vi "MC_ISM_main.vi"() -> ()   [LabVIEW 2017]
doc: "Use this template to build a user interface event handler design pattern. Use this pattern for dialog boxes and other user interfaces. You also can create and execute user-defined events that the VI can handle the same way as user interface events."
uses:
  <vilib>/Utility/error.llb/DialogType.ctl
  <vilib>/DAQmx/write.llb/DAQmx Write (Analog 1D Wfm NChan NSamp).vi
  <vilib>/DAQmx/create/channels.llb/DAQmx Create Channel (AO-Voltage-Basic).vi
  <vilib>/DAQmx/configure/timing.llb/DAQmx Timing (Sample Clock).vi
  <vilib>/DAQmx/miscellaneous.llb/DAQmx Fill In Error Info.vi
  <resource>/objmgr/daqmx.rc
panel:
  in  "Preview":enum32{"Preview"}(tab)
  out "Camera frame rate":dbl
  in  "Vertical":dbl=1024.0
  in  "Exposure time":dbl=5.0
  in  "Num of cycle":i32=2000
  out "Num of captured cycle":i32
  out "Time consumed (ms)":u32
  in  "Y size":dbl=1.0
  in  "X size":dbl=49.0
  in  "Amplitude X":dbl=0.798
  in  "Amplitude Y":dbl
  in  "Scan range (um)":dbl
  in  "Step size (um)":dbl=1.0
  in  "Multicolor":dbl=1.0
  in  "Z calibration 0.1/100nm":dbl
  in  "Slope":dbl=0.3
  in  "Dwell time":dbl=0.7
  in  "Point precision us/point":dbl=10.0
  out "Number of camera frame":dbl
  in  "First":dbl=0.3
  out "Acquisition rate":dbl
  out "Output Graph":waveform(dbl)[](graph)
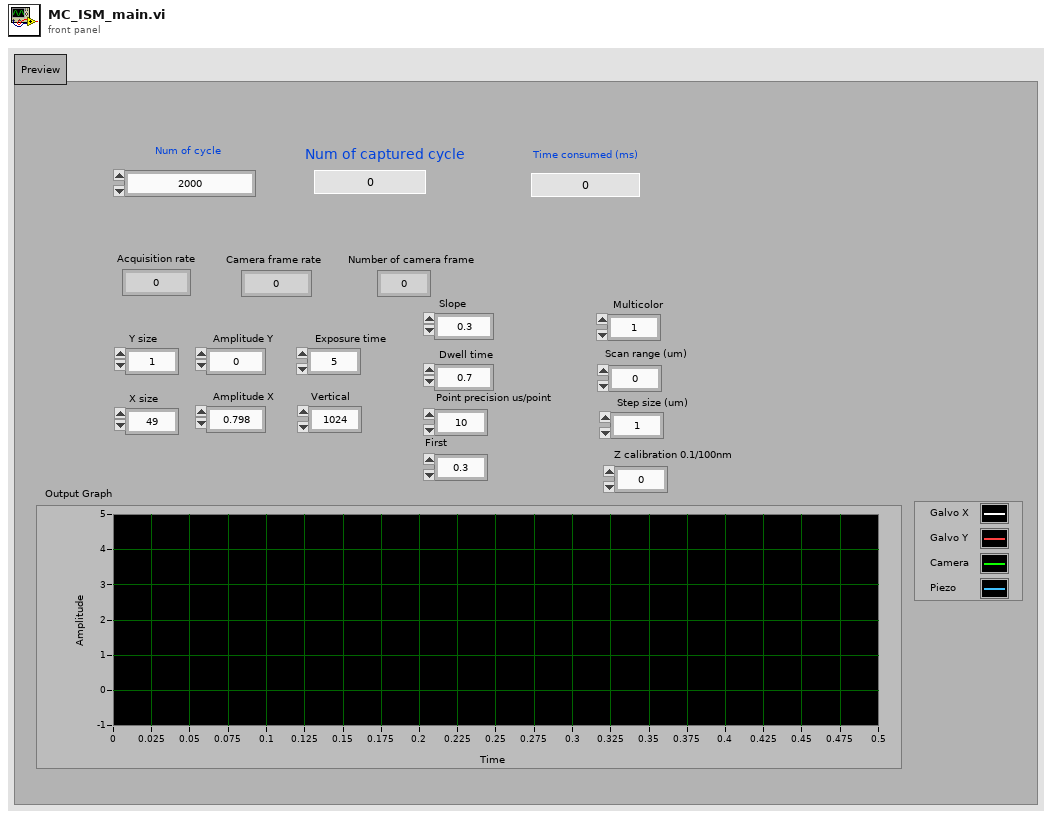
[diagram p1: front panel]
types:
  T1 = typedef "DialogType.ctl" = u16
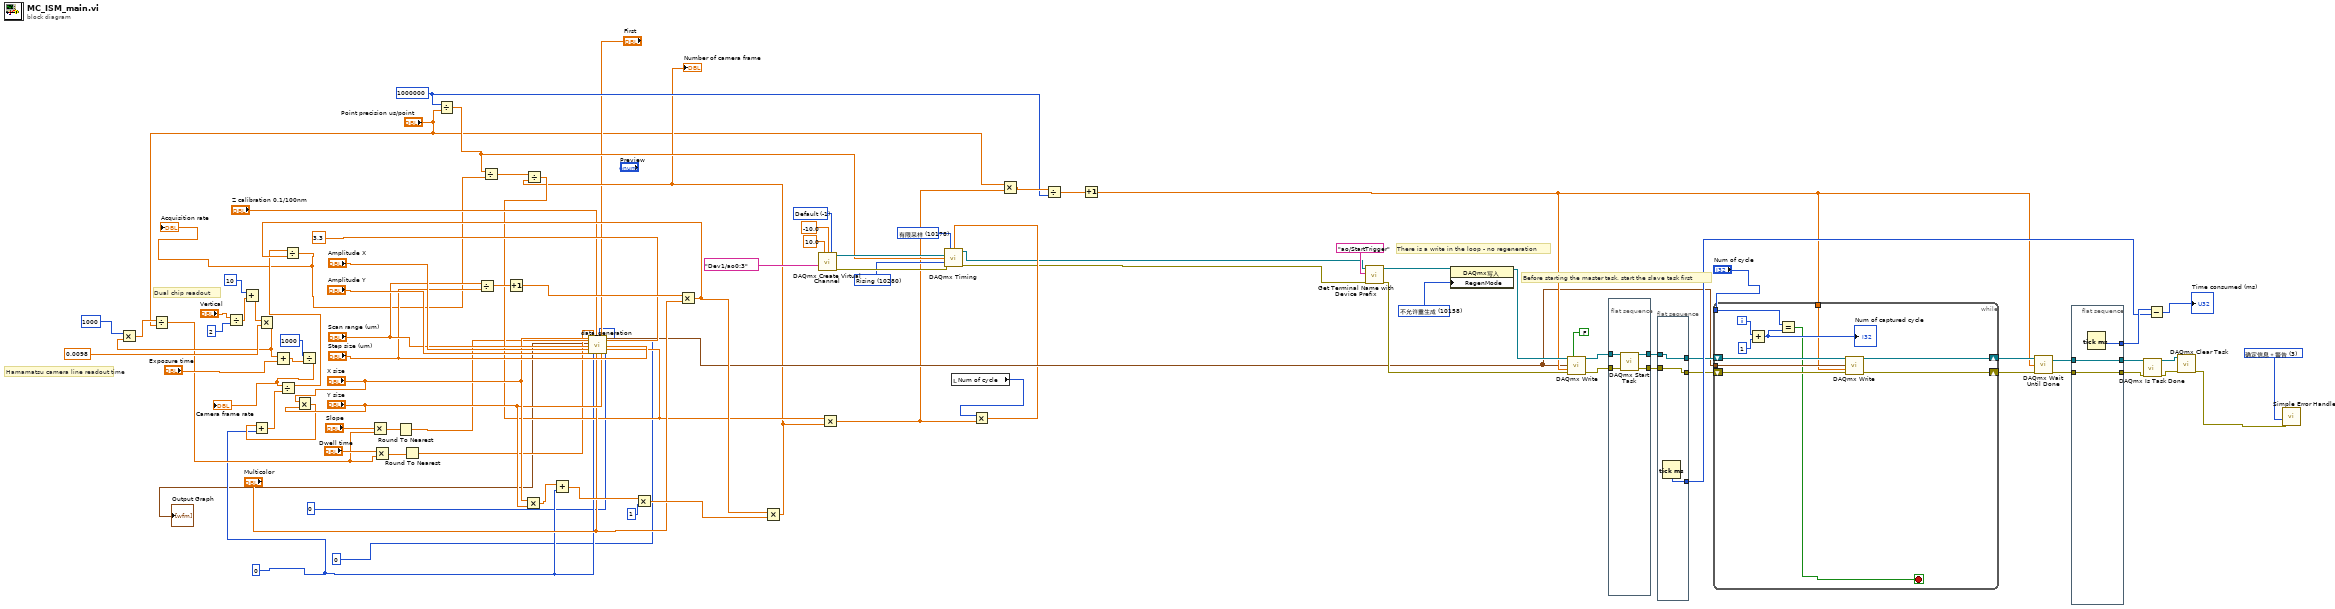
[diagram p0: block diagram]
diagram:
  w5 = 0
  w25 = 1000000
  w80 = 10158 items=["允许重生成"=10097, "不允许重生成"=10158] ("RegenMode")
  w83 = 10178 items=["有限采样"=10178, "连续采样"=10123, "硬件定时单点"=12522] ("sample mode")
  w88 = T1 3 items=["无对话框", "确定信息", "继续或停止信息", "确定信息＋警告", "继续/停止＋警告"] ("对话框类型（确定信息：1）")
  w94 = -1 items=["Default"=-1, "RSE"=10083, "Differential"=10106, "Pseudodifferential"=12529] ("output terminal configuration")
  w63 = 10280 items=["Rising"=10280, "Falling"=10171] ("active edge")
  # "Dual chip readout"
  # "Hamamatsu camera line readout time"
  # "There is a write in the loop - no regeneration"
  # "Before starting the master task, start the slave task first"
  n1 = Divide(x="Vertical", y=2) -> (x/y=w49:dbl)
  n2 = Add(x=10, y=w49) -> (x+y=w47:dbl)
  n3 = Multiply(x=w47, y=0.0098) -> (x*y=w17:dbl)
  n4 = Multiply(x=1000, y=w17) -> (x*y=w15:dbl)
  n5 = Divide(x=w15, y="Point precision us/point") -> (x/y=w13:dbl)
  n6 = Add(x=w17, y="Exposure time") -> (x+y=w51:dbl)
  n7 = Multiply(x="X size", y="Y size") -> (x*y=w40:dbl)
  n8 = Add(x=w40, y=w5) -> (x+y=w39:dbl)
  n9 = Divide(x=1000, y=w51) -> (x/y=w44:dbl)
  "Camera frame rate" <- w44
  n10 = Divide(x=w44, y=w39) -> (x/y=w42:dbl)
  n11 = Multiply(x="Slope", y=w13) -> (x*y=w12:dbl)
  n12 = Multiply(x="Dwell time", y=w13) -> (x*y=w10:dbl)
  n13 = Round To Nearest(number=w12) -> (nearest integer value=w11:dbl)
  n14 = Round To Nearest(number=w10) -> (nearest integer value=w9:dbl)
  n15 = Divide(x=w25, y="Point precision us/point") -> (x/y=w27:dbl)
  n16 = Divide(x="Scan range (um)", y="Step size (um)") -> (x/y=w57:dbl)
  n17 = Increment(x=w57) -> (x+1=w56:dbl)
  n18 = Multiply(x="X size", y="Y size") -> (x*y=w38:dbl)
  n19 = Add(x=w38, y=w5) -> (x+y=w37:dbl)
  n20 = Multiply(x=w37, y=1) -> (x*y=w55:dbl)
  n21 = Multiply(x=w56, y="Multicolor") -> (x*y=w43:dbl)
  n22 = Divide(x=w42, y=w43) -> (x/y=w2:dbl)
  "Acquisition rate" <- w2
  n23 = Divide(x=w27, y=w2) -> (x/y=w30:dbl)
  n24 = Multiply(x=w43, y=w55) -> (x*y=w21:dbl)
  "Number of camera frame" <- w21
  n25 = Divide(x=w30, y=w21) -> (x/y=w29:dbl)
  n26 = call "data_generation.vi"("X Size"="X size", "slope"=w11, "scan range (um)"="Scan range (um)", "AmplitudeX"="Amplitude X", "AmplitudeY"="Amplitude Y", "dwell time"=w9, "come back"=w5, "calibration"="Z calibration 0.1/100nm", "multicolor"="Multicolor", "zero point"=0, "first"="First", "Y size"="Y size", "AmplitudeC"=3.3, "step size (um)"="Step size (um)", "Samples per spot"=w29, "zero point 2"=0) -> ("Output Graph"=→"Output Graph":waveform(dbl)[], "XY Scan"=w23:waveform(dbl)[])  [unwired: 1 in, 1 out]
  n27 = call-poly <vilib>:"DAQmx Create Virtual Channel.vi"("maximum value"=10.0, "minimum value"=-10.0, "output terminal configuration"=w94, "physical channels"=tag "Dev1/ao0:3" ("AO channels")) -> ("task out"=w91:refnum<k21>, "error out"=w90:errorcluster)  [unwired: 10 in]
  n28 = Multiply(x=w29, y=w21) -> (x*y=w22:dbl)
  n29 = local read "Num of cycle"() -> (w62:i32)
  n30 = Multiply(x=w62, y=w22) -> (x*y=w19:dbl)
  n31 = call-poly <vilib>:"DAQmx Timing.vi"("task/channels in"=w91, "sample mode"=w83, "samples per channel"=w19, "rate"=w27, "active edge"=w63, "error in"=w90) -> ("task out"=w7:refnum<k21>, "error out"=w6:errorcluster)  [unwired: 8 in]
  n32 = Multiply(x="Point precision us/point", y=w22) -> (x*y=w26:dbl)
  n33 = Divide(x=w26, y=w25) -> (x/y=w18:dbl)
  n34 = Increment(x=w18) -> (x+1=w24:dbl)
  n35 = call "Get Terminal Name with Device Prefix.vi"("error in (no error)"=w6, "Local Terminal Name"="ao/StartTrigger" ("本地接线端名"), "task/channels in"=w7) -> ("error out"=w85:errorcluster, "task out"=w79:refnum<k21>)  [unwired: 6 in, 1 out]
  n36 = property class="DAQmx写入"(reference=w79, "RegenMode"=w80) -> (reference out=w73:refnum<k21>)  [unwired: 1 in, 1 out]
  n37 = call-poly <vilib>:"DAQmx Write.vi"("task/channels in"=w73, "auto start"=FALSE, "data"=w23, "timeout"=w24, "error in"=w85) -> ("task out"=w87:refnum<k21>, "error out"=w86:errorcluster)  [unwired: 8 in, 1 out]
  n38 = flat-sequence {
    tunnel: [w98] -> w74
    tunnel: [w97] -> w77
    tunnel: w87 -> [w96]
    tunnel: w86 -> [w95]
    frame #0 {
      n39 = call <vilib>:"DAQmx Start Task.vi"("task/channels in"=w96, "error in"=w95) -> ("task out"=w97:refnum<k21>, "error out"=w98:errorcluster)  [unwired: 12 in]
    }
  }
  n40 = flat-sequence {
    tunnel: [w101] -> w78
    tunnel: w77 -> [w100]
    tunnel: [w100] -> w76
    tunnel: [w99] -> w75
    tunnel: w74 -> [w99]
    frame #0 {
      n41 = Tick Count (ms)() -> (millisecond timer value=w101:u32)
    }
  }
  n42 = while {
    shift-right: [w108] -> w70
    shift-left: w76 -> [w109]
    shift-right: [w106] -> w69
    shift-left: w75 -> [w107]
    tunnel: "Num of cycle" -> [w110]
    tunnel: w23 -> [w104]
    tunnel: w24 -> [w103]
    i -> [w112]
    stop <- w102 stop-if-true
    n43 = Add(x=w112, y=1) -> (x+y=w105:i32)
    "Num of captured cycle" <- w105
    n44 = Equal?(x=w110, y=w105) -> (x = y?=w102:bool)
    n45 = call-poly <vilib>:"DAQmx Write.vi"("task/channels in"=w109, "data"=w104, "timeout"=w103, "error in"=w107) -> ("task out"=w108:refnum<k21>, "error out"=w106:errorcluster)  [unwired: 9 in, 1 out]
  }
  n46 = call <vilib>:"DAQmx Wait Until Done.vi"("task/channels in"=w70, "timeout (sec)"=w24, "error in"=w69) -> ("task out"=w72:refnum<k21>, "error out"=w71:errorcluster)  [unwired: 11 in]
  n47 = flat-sequence {
    tunnel: [w115] -> w82
    tunnel: w72 -> [w114]
    tunnel: [w114] -> w68
    tunnel: w71 -> [w113]
    tunnel: [w113] -> w66
    frame #0 {
      n48 = Tick Count (ms)() -> (millisecond timer value=w115:u32)
    }
  }
  n49 = call <vilib>:"DAQmx Is Task Done.vi"("task/channels in"=w68, "error in"=w66) -> ("task out"=w67:refnum<k21>, "error out"=w65:errorcluster)  [unwired: 11 in, 1 out]
  n50 = Subtract(x=w82, y=w78) -> (x-y=→"Time consumed (ms)":u32)
  n51 = call <vilib>:"DAQmx Clear Task.vi"("task in"=w67, "error in"=w65) -> ("error out"=w8:errorcluster)  [unwired: 13 in]
  n52 = call <vilib>:"Simple Error Handler.vi"("type of dialog (OK msg:1)"=w88, "error in (no error)"=w8) -> ()  [unwired: 3 in, 5 out]
